vi "ICM List Buses.vi"() -> (0 "error out":errorcluster, 3 "Buses":string[](array[string]))   [LabVIEW 2018]
doc: "ICM List Buses.vi\n\nThis VI creates a list of all the Bus child classes present in the current copy of ICM.\n\nInstrument Communication Module Version 1.0\nJuly, 2017 Original Code Consulting David Thomson\n www.originalcode.com"
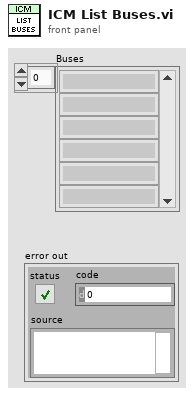
[diagram p1: front panel]
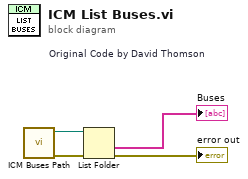
[diagram p0: block diagram]
diagram:
  n1 = call "ICM Buses Path.vi"() -> ("error out"=w3:errorcluster, "ICM Buses Path"=w4:path)  [unwired: 10 in]
  n2 = List Folder "Original Code by David Thomson"(path=w4, error in=w3) -> (folder names=→"Buses":string[], error out=→"error out":errorcluster)  [unwired: 2 in, 2 out]
